vi "serial_receiver.vi"(2 "stop receiving":bool, 4 "byte count":u32) -> (0 "error":bool, 1 "read buffer":string, 3 "return count":u32)   [LabVIEW 2014]
uses:
  <vilib>/Instr/_visa.llb/VISA Open Access Mode.ctl
panel:
  in  "Access Mode":T1 items=["VISA Defaults"=0, "Exclusive Lock"=1, "Load Configured Settings"=4]
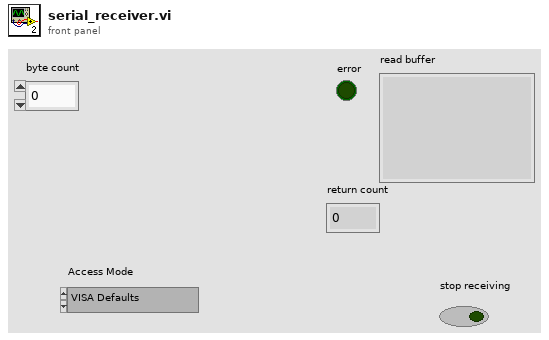
[diagram p1: front panel]
types:
  T1 = typedef "VISA Open Access Mode.ctl" = u32
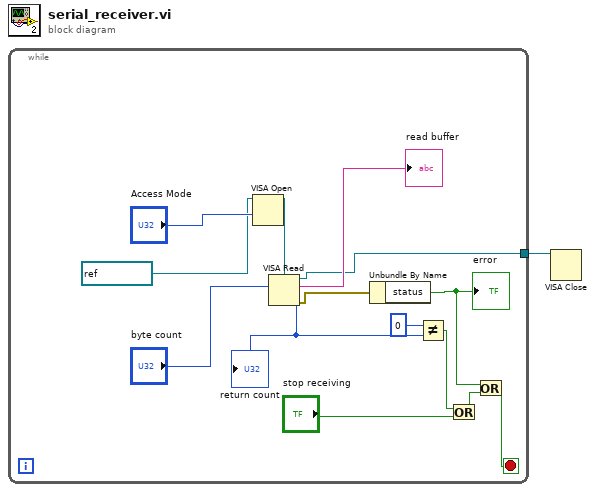
[diagram p0: block diagram]
diagram:
  n1 = while {
    tunnel: [w11] -> w1
    stop <- w3 stop-if-true
    n2 = VISA Open(access mode="Access Mode", VISA resource name=refnum<visa-resource-name> "COM2") -> (VISA resource name=w13:refnum<visa-resource-name>)  [unwired: 3 in, 1 out]
    n3 = VISA Read(VISA resource name=w13, byte count="byte count") -> (VISA resource name out=w11:refnum<visa-resource-name>, read buffer=→"read buffer":string, return count=w9:u32, error out=w6:errorcluster)  [unwired: 1 in]
    "return count" <- w9
    n4 = Unbundle By Name(w6) -> ("status"=w5:bool)
    "error" <- w5
    n5 = Not Equal?(x=u32 0, y=w9) -> (x != y?=w8:bool)
    n6 = Or(x=w8, y="stop receiving") -> (x .or. y?=w4:bool)
    n7 = Or(x=w5, y=w4) -> (x .or. y?=w3:bool)
  }
  n8 = VISA Close(VISA resource name=w1) -> ()  [unwired: 1 in, 1 out]
